vi "Draw Bullseye.vi"(5 "Step Size":i32, 6 "Bullseye Color":u32, 7 "Number of Circles":i32, 8 "error in (no error)":errorcluster, 9 "Y":i32, 10 "X":i32, 11 "Refnum in":T1) -> (0 "error out":errorcluster, 3 "Refnum out":T1)   [LabVIEW 2016]
uses:
  <vilib>/vision/Image Controls.llb/IMAQ Image.ctl
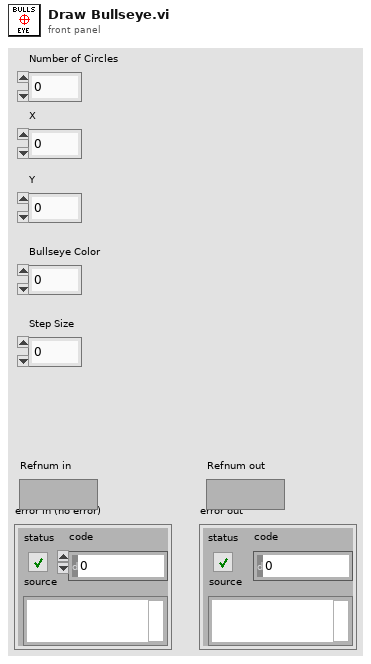
[diagram p1: front panel]
types:
  T1 = typedef "IMAQ Image.ctl" = refnum<image>
  T2 = cluster{"X Resolution":i32, "Y Resolution":i32, "X Resolution":i32, "Y Resolution":i32}
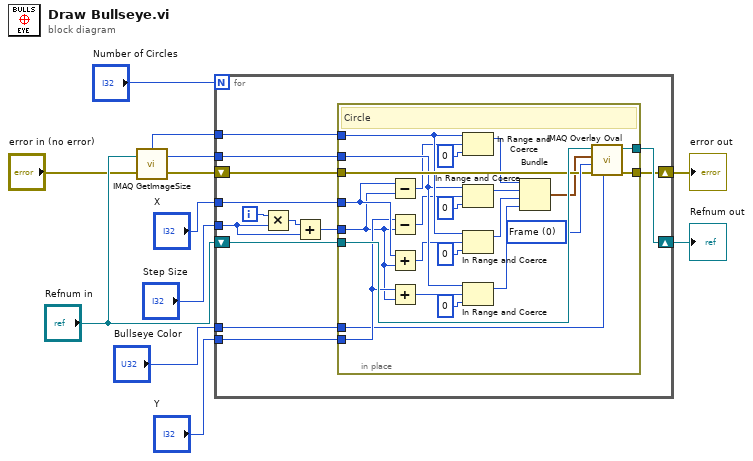
[diagram p0: block diagram]
diagram:
  n1 = call "IMAQ GetImageSize"("Image"="Refnum in", "error in (no error)"="error in (no error)") -> ("Y Resolution"=w3:i32, "X Resolution"=w4:i32, "error out"=w1:errorcluster)  [unwired: 2 in]
  n2 = for {
    N: "Number of Circles" -> [_]
    tunnel: w4 -> [w21]
    tunnel: w3 -> [w20]
    tunnel: "X" -> [w19]
    tunnel: "Y" -> [w18]
    shift-right: [w24] -> w6
    shift-left: "Refnum in" -> [w25]
    shift-right: [w22] -> w7
    shift-left: w1 -> [w23]
    tunnel: "Bullseye Color" -> [w14]
    tunnel: "Step Size" -> [w13]
    i -> [w17]
    n3 = Multiply(x=w17, y=w13) -> (x*y=w16:i32)
    n4 = Add(x=w16, y=w13) -> (x+y=w15:i32)
    n5 = in-place {
      in-place-border: w25 -> [w49]
      in-place-border: [w47] -> w24
      in-place-border: w23 -> [w46]
      in-place-border: [w45] -> w22
      in-place-border: w21 -> [w39]
      in-place-border: w20 -> [w36]
      in-place-border: w19 -> [w33]
      in-place-border: w18 -> [w32]
      in-place-border: w15 -> [w27]
      in-place-border: w14 -> [w26]
      w48 = u32 0 items=["Frame", "Fill"] ("Drawing Mode (Frame)")
      # "Circle"
      n6 = Subtract(x=w33, y=w27) -> (x-y=w31:i32)
      n7 = Subtract(x=w32, y=w27) -> (x-y=w29:i32)
      n8 = Add(x=w33, y=w27) -> (x+y=w30:i32)
      n9 = Add(x=w32, y=w27) -> (x+y=w28:i32)
      n10 = In Range and Coerce(upper limit=w39, x=w31, lower limit=0) -> (coerced(x)=w43:i32)  [unwired: 1 out]
      n11 = In Range and Coerce(upper limit=w36, x=w29, lower limit=0) -> (coerced(x)=w41:i32)  [unwired: 1 out]
      n12 = In Range and Coerce(upper limit=w39, x=w30, lower limit=0) -> (coerced(x)=w38:i32)  [unwired: 1 out]
      n13 = In Range and Coerce(upper limit=w36, x=w28, lower limit=0) -> (coerced(x)=w35:i32)  [unwired: 1 out]
      n14 = Bundle("X Resolution"=w43, "Y Resolution"=w41, "X Resolution"=w38, "Y Resolution"=w35) -> (w34:T2)  [unwired: 1 in]
      n15 = call "IMAQ Overlay Oval"("Color"=w26, "error in (no error)"=w46, "Drawing Mode (Frame)"=w48, "Bounding Rectangle"=w34, "Image"=w49) -> ("error out"=w45:errorcluster, "Image Out"=w47:T1)  [unwired: 5 in]
    }
  }
  "error out" <- w7
  "Refnum out" <- w6
